vi "Func Processor for Events.vi"(6 "Math Assign In":string[](array[string]), 8 "Triggering Math In":string[](array[string]), 9 "Fn Arg Cnt":string[](array[string]), 10 "Functions Definition":string[][](table), 11 "Total Function Definitions":i32) -> (1 "Math Assign Out":string[](array[string]), 3 "Triggering Math Out":string[](array[string]))   [LabVIEW 2014]
panel:
  out "Fn-Math":string[](array[string])
  out "Fn Name":string[](array[string])
  # "External Inputs"
  # "Intermediate variables"
  # "Outputs"
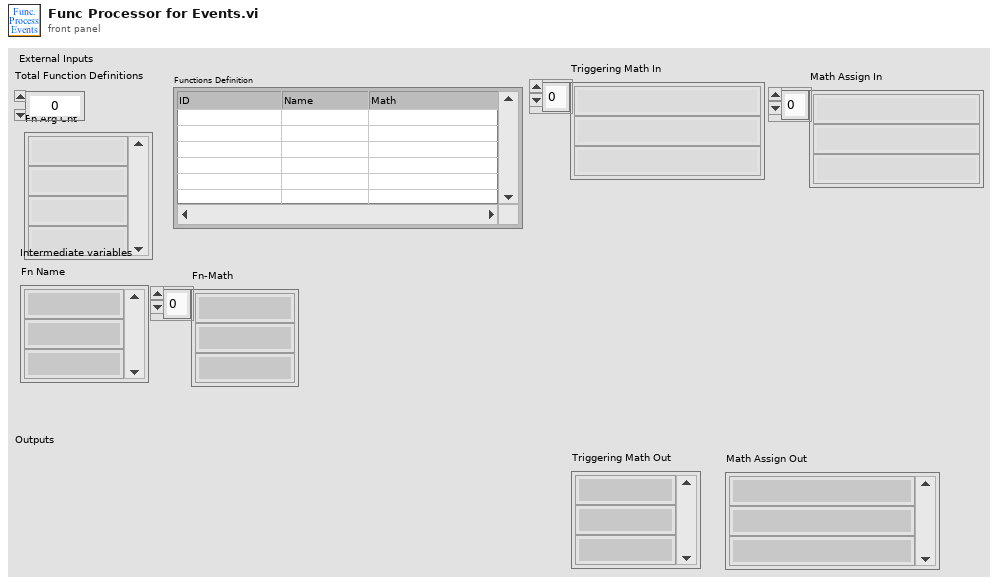
[diagram p1: front panel]
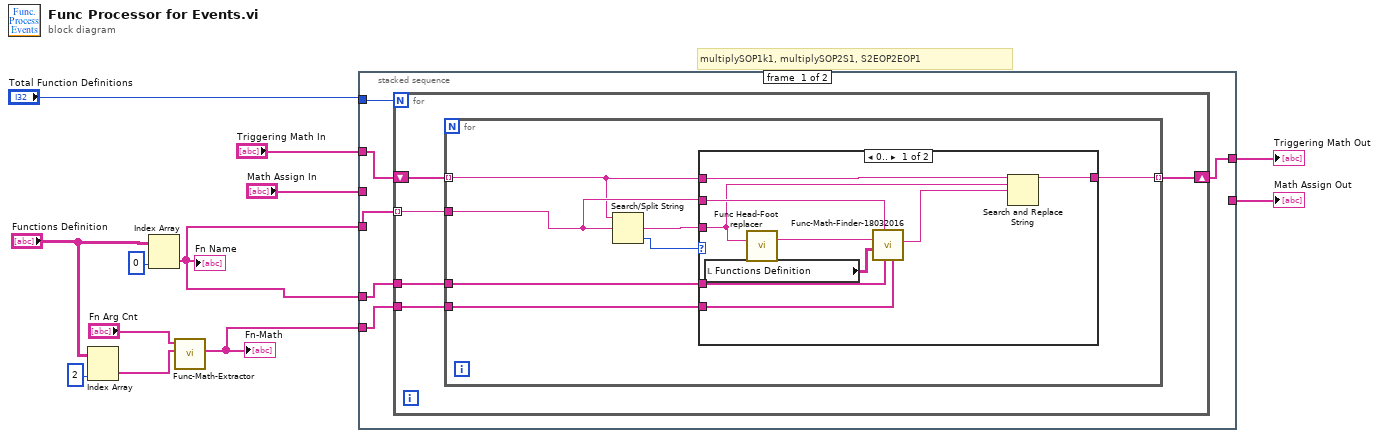
[diagram p0: block diagram]
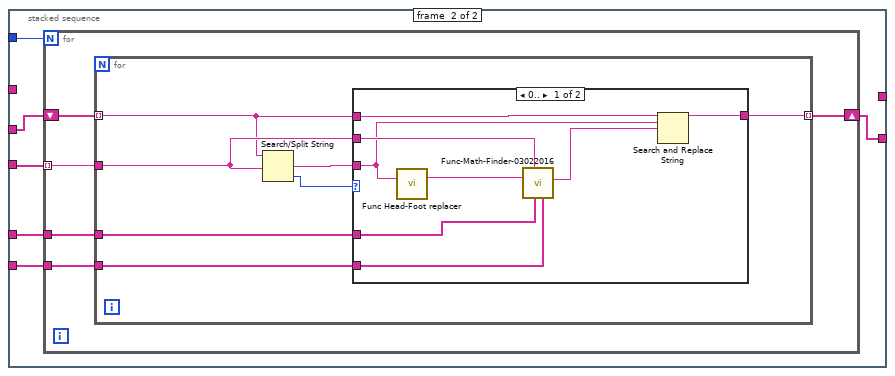
[diagram p3: hidden frame]
diagram:
  # "multiplySOP1k1, multiplySOP2S1, S2EOP2EOP1"
  n1 = Index Array(array="Functions Definition", index (col)=2 ("disabled index (col)")) -> (element=w8:string[])  [unwired: 1 in]
  n2 = Index Array(array="Functions Definition", index (col)=0 ("disabled index (col)")) -> (element=w1:string[])  [unwired: 1 in]
  "Fn Name" <- w1
  n3 = call "Func-Math-Extractor.vi"("Fn Math"=w8, "Fn Arg Cnt"="Fn Arg Cnt") -> ("Fn-Math"=w2:string[])  [unwired: 9 in]
  "Fn-Math" <- w2
  n4 = stacked-sequence {
    tunnel: "Total Function Definitions" -> [w18 w46]
    tunnel: w1 -> [w17 w45]
    tunnel: "Triggering Math In" -> [w16 _]
    tunnel: [w15 _] -> w6
    tunnel: "Math Assign In" -> [_ w44]
    tunnel: [_ w43] -> w3
    tunnel: w2 -> [w13 w42]
    tunnel: w1 -> [w14 w41]
    frame #0 {
      n5 = for {
        N: w18 -> [_]
        tunnel: w17 -> [w22] mode=indexing
        shift-right: [w21] -> w15
        shift-left: w16 -> [w23]
        tunnel: w14 -> [w20]
        tunnel: w13 -> [w19]
        n6 = for {
          tunnel: w23 -> [w27] mode=indexing
          tunnel: w22 -> [w29]
          tunnel: [w26] -> w21 mode=indexing
          tunnel: w20 -> [w25]
          tunnel: w19 -> [w24]
          n7 = Search/Split String(string=w27, search string/char (-)=w29) -> (match + rest of string=w30:string, offset of match=w28:i32)  [unwired: 1 in, 1 out]
          n8 = case shown="0.." w28 {
            tunnel: w30 -> [w36 _]
            tunnel: w29 -> [w38 _]
            tunnel: w27 -> [w37 w40]
            tunnel: [w34 w40] -> w26
            tunnel: w25 -> [w33 _]
            tunnel: w24 -> [w32 _]
            frame 0.. {
              n9 = local read "Functions Definition"() -> (w31:string[][])
              n10 = call "Func Head-Foot replacer.vi"("Function in"=w36) -> ("Function in Out"=w39:string)  [unwired: 12 in, 2 out]
              n11 = call "Func-Math-Finder-18032016.vi"("All Fn-Math"=w32, "All Fn Name"=w33, "Func Name"=w38, "Functions Definition"=w31, "Get Tagged String"=w39) -> ("Expression"=w35:string)  [unwired: 4 in, 2 out]
              n12 = Search and Replace String(input string=w37, search string=w36, replace string=w35) -> (result string=w34:string)  [unwired: 5 in, 3 out]
            }
            frame -1, Default {
            }
          }
        }
      }
    }
    frame #1 {
      n13 = for {
        N: w46 -> [_]
        tunnel: w45 -> [w50] mode=indexing
        shift-right: [w49] -> w43
        shift-left: w44 -> [w51]
        tunnel: w42 -> [w48]
        tunnel: w41 -> [w47]
        n14 = for {
          tunnel: w51 -> [w55] mode=indexing
          tunnel: w50 -> [w57]
          tunnel: [w54] -> w49 mode=indexing
          tunnel: w48 -> [w53]
          tunnel: w47 -> [w52]
          n15 = Search/Split String(string=w55, search string/char (-)=w57) -> (match + rest of string=w58:string, offset of match=w56:i32)  [unwired: 1 in, 1 out]
          n16 = case shown="0.." w56 {
            tunnel: w58 -> [w63 _]
            tunnel: w57 -> [w65 _]
            tunnel: w55 -> [w64 w67]
            tunnel: [w61 w67] -> w54
            tunnel: w53 -> [w60 _]
            tunnel: w52 -> [w59 _]
            frame 0.. {
              n17 = call "Func Head-Foot replacer.vi"("Function in"=w63) -> ("Function in Out"=w66:string)  [unwired: 12 in, 2 out]
              n18 = call "Func-Math-Finder-03022016.vi"("All Fn-Math"=w60, "All Fn Name"=w59, "Func Name"=w65, "Get Tagged String"=w66) -> ("Expression"=w62:string)  [unwired: 5 in, 2 out]
              n19 = Search and Replace String(input string=w64, search string=w63, replace string=w62) -> (result string=w61:string)  [unwired: 5 in, 3 out]
            }
            frame -1, Default {
            }
          }
        }
      }
    }
  }
  "Triggering Math Out" <- w6
  "Math Assign Out" <- w3
